vi "PXI-Max Aggregate Sampling Rate.vi"(0 "task in":refnum<k21>, 2 "Mode":enum16{"AO", "AI", "DO", "DI"}(ring), 7 "Agg Sampling Rate":dbl, 11 "error in (no error)":errorcluster) -> (4 "task out":refnum<k21>, 8 "MaxRate":dbl, 15 "error out":errorcluster)   [LabVIEW 2020]
uses:
  <resource>/objmgr/daqmx.rc
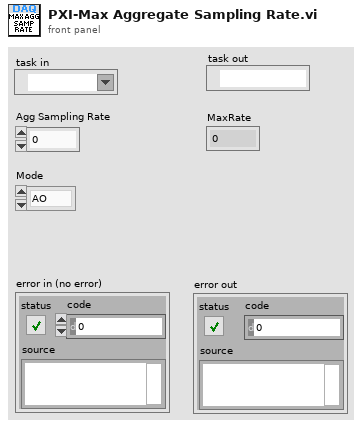
[diagram p1: front panel]
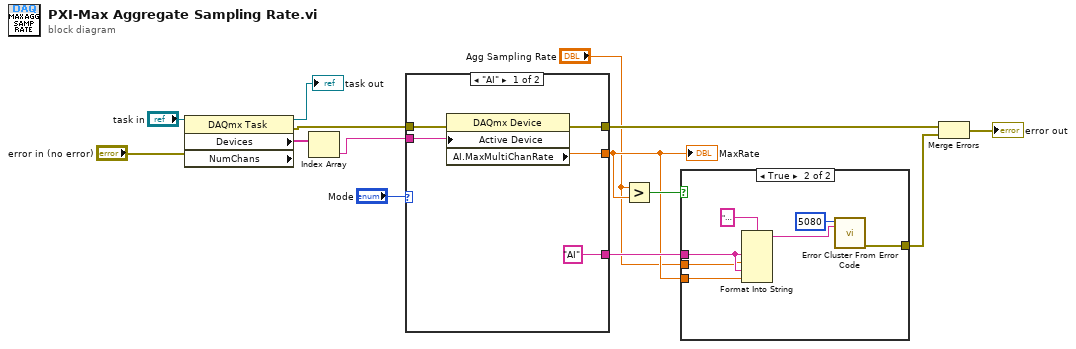
[diagram p0: block diagram]
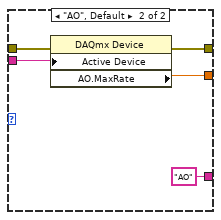
[diagram p2: hidden frame]
diagram:
  n1 = property class="DAQmx Task" props=["Devices", "NumChans"](reference="task in", error in="error in (no error)") -> (reference out=→"task out":refnum<k21>, error out=w11:errorcluster, "Devices"=w14:tag[])  [unwired: 1 out]
  n2 = Index Array(array=w14) -> (element=w13:tag)  [unwired: 1 in]
  n3 = case shown="\"AI\"" "Mode" {
    tunnel: w13 -> [w19 w24]
    tunnel: w11 -> [w18 w23]
    tunnel: [w17 w22] -> w9
    tunnel: [w16 w21] -> w2
    tunnel: ["AI" "AO"] -> w3
    frame "AI" {
      n4 = property class="DAQmx Device"(error in=w18, "Active Device"=w19) -> (error out=w17:errorcluster, "AI.MaxMultiChanRate"=w16:dbl)  [unwired: 1 in, 1 out]
    }
    frame "AO", Default {
      n5 = property class="DAQmx Device"(error in=w23, "Active Device"=w24) -> (error out=w22:errorcluster, "AO.MaxRate"=w21:dbl)  [unwired: 1 in, 1 out]
    }
  }
  "MaxRate" <- w2
  n6 = Greater?(x="Agg Sampling Rate", y=w2) -> (0:w7:bool)
  n7 = case shown="True" w7 {
    tunnel: [_ w30] -> w5
    tunnel: w3 -> [_ w27]
    tunnel: w2 -> [_ w26]
    tunnel: "Agg Sampling Rate" -> [_ w25]
    frame False {
    }
    frame True {
      n8 = Format Into String(format string="Aggregate %s sampling rate  = %#g Hz\nMaximum %s sampling rate  = %#g Hz", w27, w25, w27, w26) -> (resulting string=w28:string)  [unwired: 2 in, 1 out]
      n9 = call <vilib>:"Error Cluster From Error Code.vi"("error message (\"\")"=w28, "error code (0)"=5080) -> ("error out"=w30:errorcluster)  [unwired: 7 in]
    }
  }
  n10 = Merge Errors(w9, w5) -> (→"error out":errorcluster)
